vi "Module Loop.vi"(8 "error in (no error)":errorcluster, 11 "DAQmxDI in":refnum<class " DAQmxDI Port.lvclass">) -> (0 "error out":errorcluster, 3 "DAQmxDI out":refnum<class " DAQmxDI Port.lvclass">)   [LabVIEW 2020, in " DAQmxDI Port.lvclass"]
uses:
   DAQmxDI Port.lvclass
   DAQmxDI Port.lvclass/ DAQmxDI Port.ctl
  Volatus/Module/Module.lvclass
  C:/dev/lv20CE/relink/lv-volatus/Volatus/Module/Module.lvclass
  C:/dev/lv20CE/relink/lv-volatus/VolatusDAQ/DAQmxDI Port/ DAQmxDI Port.lvclass
  Volatus/MessageQ/MessageQ.lvclass
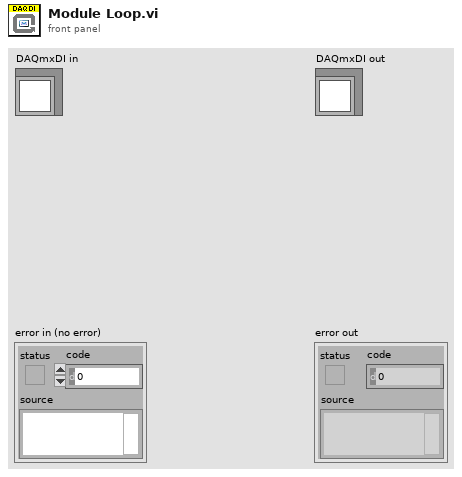
[diagram p1: front panel]
types:
  T1 = enum32{"Invalid", "Standard", "Closed", "Hidden", "Minimized", "Maximized"}
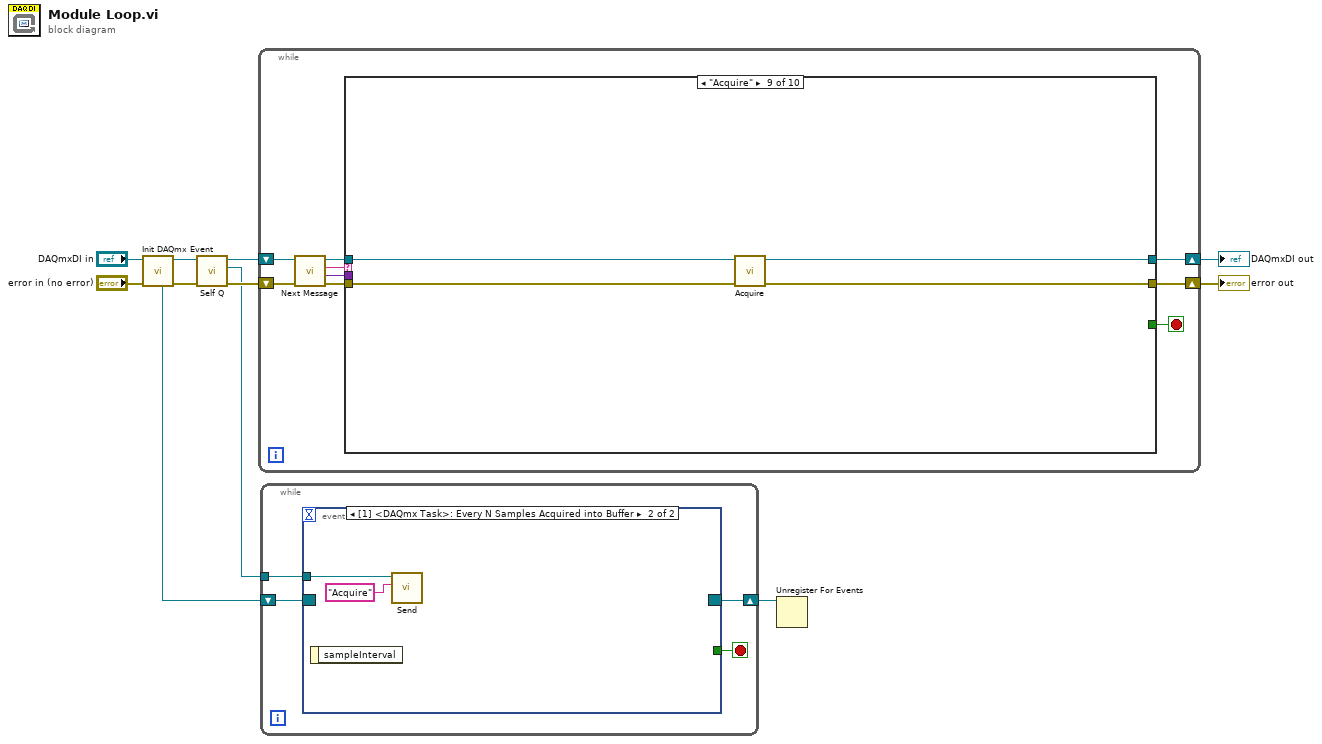
[diagram p0: block diagram]
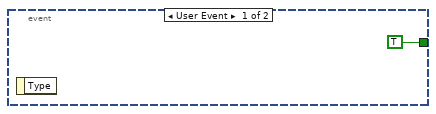
[diagram p2: hidden frame]
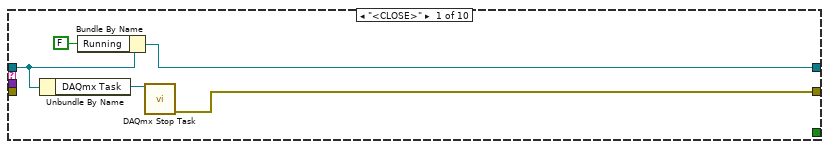
[diagram p3: hidden frame]
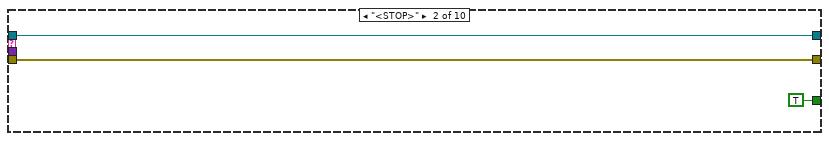
[diagram p4: hidden frame]
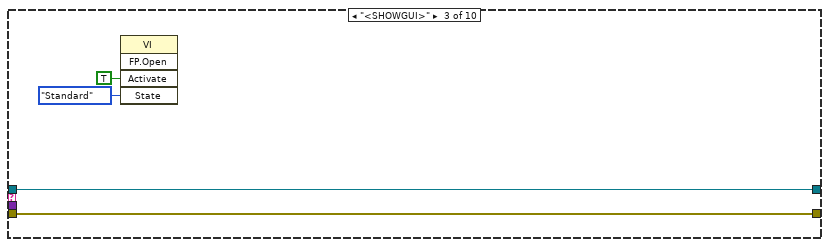
[diagram p5: hidden frame]
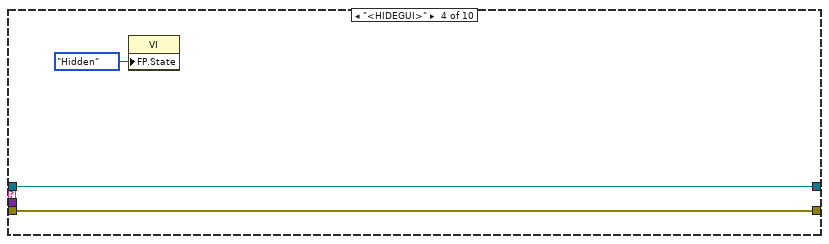
[diagram p6: hidden frame]
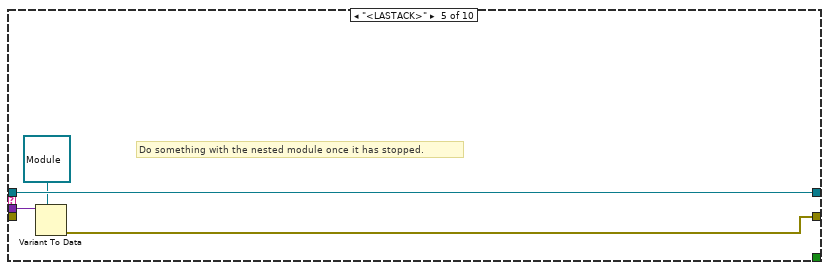
[diagram p7: hidden frame]
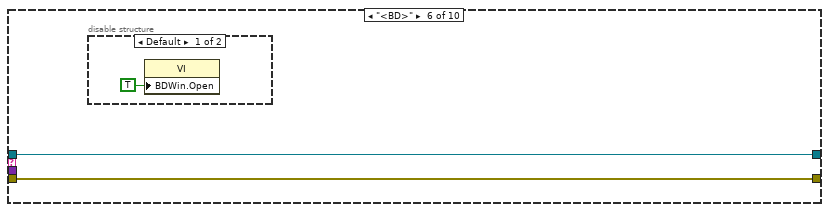
[diagram p8: hidden frame]
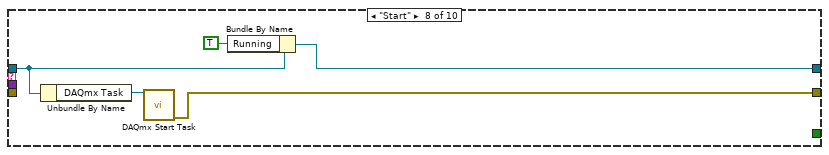
[diagram p11: hidden frame]
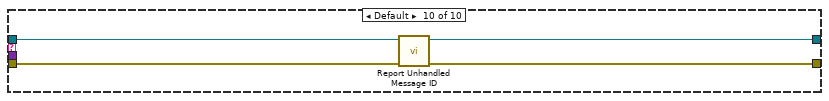
[diagram p12: hidden frame]
diagram:
  n1 = call "Init DAQmx Event.vi"("error in (no error)"="error in (no error)", "DAQmxDI in"="DAQmxDI in") -> ("error out"=w6:errorcluster, "DAQmxDI out"=w4:refnum<class " DAQmxDI Port.lvclass">, "Event Reg"=w3:refnum<event-registration>)  [unwired: 7 in]
  n2 = call "Self Q.vi"("Module in"=w4) -> ("Self Q"=w1:refnum<class "MessageQ.lvclass">, "Module out"=w2:refnum<class " DAQmxDI Port.lvclass">)  [unwired: 9 in]
  n3 = while {
    shift-right: [w14] -> w9
    shift-left: w2 -> [w19]
    shift-right: [w13] -> w8
    shift-left: w6 -> [w18]
    stop <- w12 stop-if-true
    n4 = call "Next Message.vi"("error in (no error)"=w18, "Module in"=w19) -> ("error out"=w17:errorcluster, "Data"=w11:variant, "ID"=w16:string, "Module out"=w15:refnum<class " DAQmxDI Port.lvclass">)  [unwired: 6 in]
    n5 = case shown="\"Acquire\"" w16 {
      tunnel: w17 -> [_ w26 w30 w33 _ w39 w43 _ w52 w56]
      tunnel: w15 -> [w23 w27 w31 w34 w38 w40 w42 w48 w50 w54]
      tunnel: [w21 w27 w31 w34 w38 w40 w42 w45 w49 w53] -> w14
      tunnel: [w22 w26 w30 w33 w35 w39 w43 w46 w51 w55] -> w13
      tunnel: [_ TRUE _ _ _ _ _ _ _ _] -> w12
      tunnel: w11 -> [_ _ _ _ w37 _ _ _ _ _]
      frame "<CLOSE>" {
        n6 = Unbundle By Name(w23) -> ("DAQmx Task"=w24:refnum<k21>)
        n7 = Bundle By Name(cluster=w23, "Running"=FALSE) -> (w21:refnum<class " DAQmxDI Port.lvclass">)
        n8 = call <vilib>:"DAQmx Stop Task.vi"("task/channels in"=w24) -> ("error out"=w22:errorcluster)  [unwired: 13 in, 1 out]
      }
      frame "<STOP>" {
      }
      frame "<SHOWGUI>" {
        n9 = invoke class="VI" method="FP.Open"("Activate"=TRUE ("Activate?"), "State"=T1."Standard") -> ()  [unwired: 3 in, 5 out]
      }
      frame "<HIDEGUI>" {
        n10 = property class="VI"("FP.State"=T1."Hidden" ("Front Panel Window:State")) -> ()  [unwired: 2 in, 2 out]
      }
      frame "<LASTACK>" {
        # "Do something with the nested module once it has stopped."
        n11 = Variant To Data(type=refnum<class "Module.lvclass"> refnum ("Volatus:Module"), Variant=w37) -> (error out=w35:errorcluster)  [unwired: 1 in, 1 out]
      }
      frame "<BD>" {
        n12 = disable-structure shown="Default" {
          frame condition #0 (active) {
            n13 = property class="VI"("BDWin.Open"=TRUE ("Block Diagram Window:Open")) -> ()  [unwired: 2 in, 2 out]
          }
          frame condition #1 {
          }
        }
      }
      frame "<TIMEOUT>" {
        # "No message for this module was received in time"
      }
      frame "Start" {
        n14 = Unbundle By Name(w48) -> ("DAQmx Task"=w47:refnum<k21>)
        n15 = call <vilib>:"DAQmx Start Task.vi"("task/channels in"=w47) -> ("error out"=w46:errorcluster)  [unwired: 13 in, 1 out]
        n16 = Bundle By Name(cluster=w48, "Running"=TRUE) -> (w45:refnum<class " DAQmxDI Port.lvclass">)
      }
      frame "Acquire" {
        n17 = call "Acquire.vi"("error in (no error)"=w52, "DAQmxDI in"=w50) -> ("error out"=w51:errorcluster, "DAQmxDI out"=w49:refnum<class " DAQmxDI Port.lvclass">)  [unwired: 8 in]
      }
      frame Default {
        n18 = call "Report Unhandled Message ID.vi"("error in (no error)"=w56, "Module in"=w54) -> ("error out"=w55:errorcluster, "Module out"=w53:refnum<class " DAQmxDI Port.lvclass">)  [unwired: 8 in]
      }
    }
  }
  "error out" <- w8
  "DAQmxDI out" <- w9
  n19 = while {
    tunnel: w1 -> [w59]
    shift-right: [w58] -> w7
    shift-left: w3 -> [w60]
    stop <- w57 stop-if-true
    n20 = event shown="[1] <DAQmx Task>: Every N Samples Acquired into Buffer" {
      selector: w60 -> [_ _]
      dyn-events: [_ _] -> w58
      timeout: _ -> [_ _]
      tunnel: w59 -> [_ w63]
      tunnel: [TRUE _] -> w57
      event User Event {
        n21 = event-data() -> ()  [unwired: 1 in, 1 out]
      }
      event Every N Samples Acquired into Buffer {
        n22 = event-data() -> ()  [unwired: 1 in, 1 out]
        n23 = call "Send.vi"("ID"="Acquire", "MessageQ in"=w63) -> ()  [unwired: 8 in, 2 out]
      }
    }
  }
  n24 = Unregister For Events(event registration refnum=w7) -> ()  [unwired: 1 in, 1 out]
